vi "execute.vi"(0 "HGF_ThreadTask":refnum<class "HGF_ThreadTask.lvclass">, 5 "error in (no error)":errorcluster, 8 "HGF_ThreadWorker":refnum<class "HGF_ThreadWorker.lvclass">) -> (10 "dup HGF_ThreadWorker":refnum<class "HGF_ThreadWorker.lvclass">, 14 "dup HGF_ThreadTask":refnum<class "HGF_ThreadTask.lvclass">, 19 "error out":errorcluster)   [LabVIEW 2014, in "HGF_BaseClasses.lvlib" / "HGF_ThreadTask.lvclass"]
uses:
  HGF_ThreadTask.lvclass
  HGF_ThreadWorker/HGF_ThreadWorker.lvclass
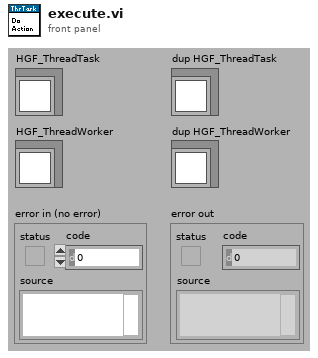
[diagram p1: front panel]
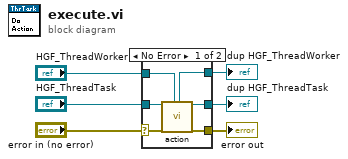
[diagram p0: block diagram]
diagram:
  n1 = case shown="No Error" "error in (no error)" {
    selector: "error in (no error)" -> [w10 w15]
    tunnel: [w9 w15] -> w5
    tunnel: [w11 w14] -> w3
    tunnel: "HGF_ThreadTask" -> [w12 w14]
    tunnel: "HGF_ThreadWorker" -> [w8 w13]
    tunnel: [w7 w13] -> w1
    frame No Error {
      n2 = call-dynamic "action.vi"("HGF_ThreadTask"=w12, "error in (no error)"=w10, "HGF_ThreadWorker"=w8) -> ("dup HGF_ThreadWorker"=w7:refnum<class "HGF_ThreadWorker.lvclass">, "dup HGF_ThreadTask"=w11:refnum<class "HGF_ThreadTask.lvclass">, "error out"=w9:errorcluster)  [unwired: 14 out]
    }
    frame Error {
    }
  }
  "error out" <- w5
  "dup HGF_ThreadTask" <- w3
  "dup HGF_ThreadWorker" <- w1
